vi "Wczytanie_nazw_kanalow_AI.vi"(8 "error in (no error)":errorcluster, 10 "AiParamsIn":T1[](array[typedef]) {"Numer" min=1 max=8 step=1}, 11 "AIcontrol refs":refnum<vi>[](array[refnum])) -> (0 "error out":errorcluster, 2 "AiParamsOut":T1[](array[typedef]) {"Numer" min=1 max=8 step=1})   [LabVIEW 2013]
uses:
  Kontrolki/GUI/AI_parametry.ctl
  Kontrolki/GUI/AI_wartosc.ctl
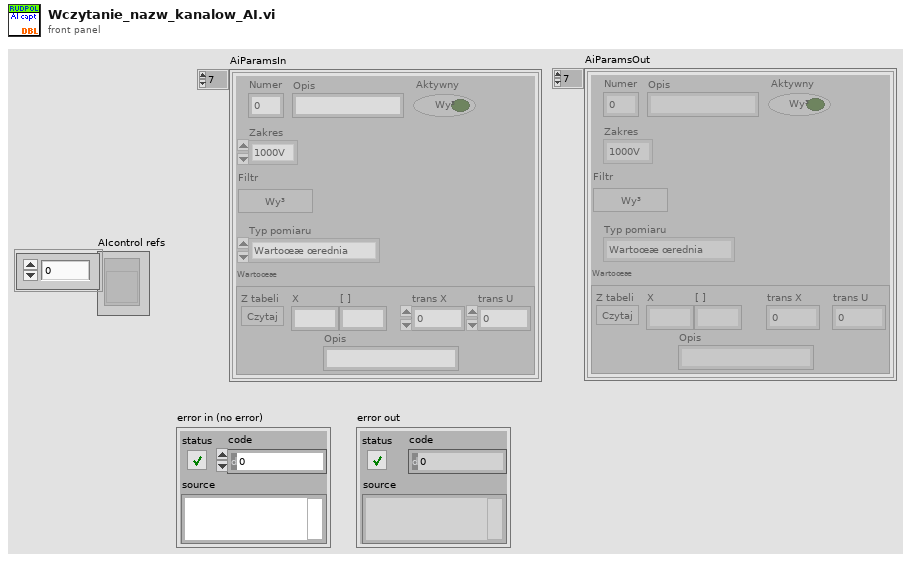
[diagram p1: front panel]
types:
  T1 = typedef "AI_parametry.ctl" = cluster{"Numer":u8, "Opis":string, "Zakres":enum16{"1000V", "300V", "30V", "3V", "0,3V"}, "Filtr":bool, "Typ pomiaru":enum16{"Wartoœæ œrednia", "Œrednia wyprostowana", "Wartoœæ skuteczna"}, "Aktywny":bool, "Wartoœæ":T2}
  T2 = typedef "AI_wartosc.ctl" = cluster{"X":string, "[ ]":string, "trans X":dbl, "trans U":dbl, "Z tabeli":bool, "Opis":string}
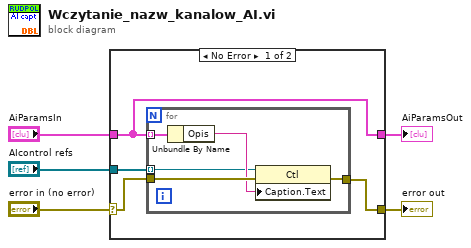
[diagram p0: block diagram]
diagram:
  n1 = case shown="No Error" "error in (no error)" {
    selector: "error in (no error)" -> [w8 w16]
    tunnel: [w7 w16] -> w4
    tunnel: "AiParamsIn" -> [w6 w15]
    tunnel: "AIcontrol refs" -> [w9 _]
    tunnel: [w6 w15] -> w2
    frame No Error {
      n2 = for {
        tunnel: w6 -> [w14] mode=indexing
        tunnel: w8 -> [w13]
        tunnel: w9 -> [w10] mode=indexing
        tunnel: [w11] -> w7
        n3 = Unbundle By Name(w14) -> ("Opis"=w12:string)
        n4 = property class="Ctl"(reference=w10, error in=w13, "Caption.Text"=w12) -> (error out=w11:errorcluster)  [unwired: 1 out]
      }
    }
    frame Error {
    }
  }
  "error out" <- w4
  "AiParamsOut" <- w2
